vi "Get Dependencies.vi"(8 "error in (no error)":errorcluster, 11 "Instrument in":refnum<class "Instrument.lvclass">) -> (0 "error out":errorcluster, 2 "Dependencies":T1, 3 "Instrument out":refnum<class "Instrument.lvclass">)   [LabVIEW 2019, in "Instrument.lvlib" / "Instrument.lvclass"]
uses:
  Instrument.lvclass
  Typedefs/Dependencies--Cluster.ctl
  <userlib>/LevyLab/Configuration/Configuration.lvclass
  subsystems/HAL/HAL.lvclass
  subsystems/API/API.lvclass
  <userlib>/LevyLab/Logger.PGSQL/Logger.PGSQL/Logger.PGSQL.lvclass
  <userlib>/LevyLab/Logger.Error/Logger.Error/Logger.Error.lvclass
  <userlib>/LevyLab/RemoteControl/RemoteControl/RemoteControl.lvclass
  C:/Program Files (x86)/National Instruments/LabVIEW 2019/vi.lib/JKI/JKI SMO/SMO/SMO.lvclass
  Instrument.lvclass/Instrument.ctl
  Typedefs/Dependencies--Enum.ctl
  <vilib>/JKI/JKI SMO/SMO/SMO.lvclass
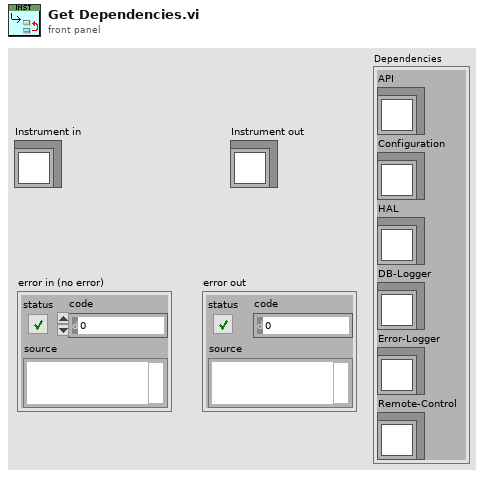
[diagram p1: front panel]
types:
  T1 = typedef "Instrument.lvlib/Instrument.lvclass/Dependencies--Cluster.ctl" = cluster{"API":refnum<class "API.lvclass">, "Configuration":refnum<class "Configuration.lvclass">, "HAL":refnum<class "HAL.lvclass">, "DB-Logger":refnum<class "Logger.PGSQL.lvclass">, "Error-Logger":refnum<class "Logger.Error.lvclass">, "Remote-Control":refnum<class "RemoteControl.lvclass">}
  T2 = typedef "Instrument.lvlib/Instrument.lvclass/Dependencies--Enum.ctl" = enum16{"API", "Configuration", "HAL", "DB-Logger", "Error-Logger", "Remote-Control"}
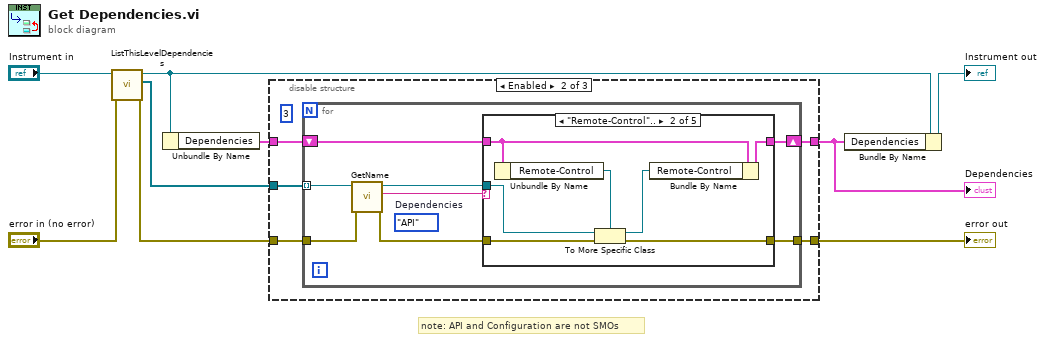
[diagram p0: block diagram]
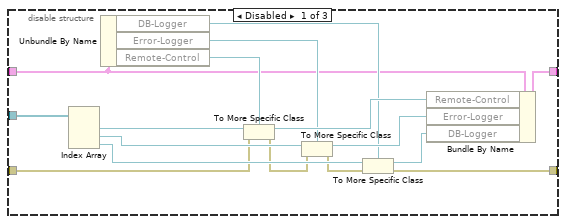
[diagram p2: hidden frame]
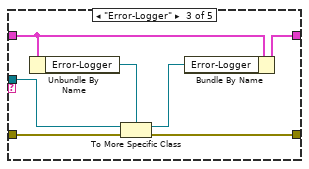
[diagram p4: hidden frame]
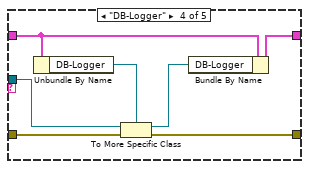
[diagram p5: hidden frame]
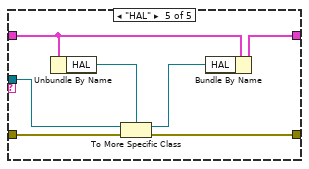
[diagram p6: hidden frame]
diagram:
  # "note: API and Configuration are not SMOs"
  n1 = call <vilib>:"ListThisLevelDependencies.vi"("error in (no error)"="error in (no error)", "SMO in"="Instrument in") -> ("error out"=w7:errorcluster, "[My Dependencies]"=w2:refnum<class "SMO.lvclass">[], "SMO out"=w5:refnum<class "Instrument.lvclass">)  [unwired: 7 in]
  n2 = Unbundle By Name(w5) -> ("Dependencies"=w4:T1)
  n3 = disable-structure shown="Enabled" {
    disable-tunnel: w7 -> [w20 w29 w69]
    disable-tunnel: w4 -> [w16 w26 w70]
    disable-tunnel: [w15 w28 w69] -> w3
    disable-tunnel: w2 -> [w14 w30 _]
    disable-tunnel: [w13 w27 w70] -> w1
    frame Disabled {
      n4 = Index Array(array=w14) -> (element #1=w25:refnum<class "SMO.lvclass">, element #2=w23:refnum<class "SMO.lvclass">, element #3=w22:refnum<class "SMO.lvclass">)  [unwired: 3 in]
      n5 = Unbundle By Name(w16) -> ("DB-Logger"=w17:refnum<class "Logger.PGSQL.lvclass">, "Error-Logger"=w18:refnum<class "Logger.Error.lvclass">, "Remote-Control"=w19:refnum<class "RemoteControl.lvclass">)
      n6 = To More Specific Class(target class=w19, reference=w25, error in=w20) -> (specific class reference=w24:refnum<class "RemoteControl.lvclass">, error out=w10:errorcluster)
      n7 = To More Specific Class(target class=w18, reference=w23, error in=w10) -> (specific class reference=w21:refnum<class "Logger.Error.lvclass">, error out=w11:errorcluster)
      n8 = To More Specific Class(target class=w17, reference=w22, error in=w11) -> (specific class reference=w12:refnum<class "Logger.PGSQL.lvclass">, error out=w15:errorcluster)
      n9 = Bundle By Name(cluster=w16, "Remote-Control"=w24, "Error-Logger"=w21, "DB-Logger"=w12) -> (w13:T1)
    }
    frame Enabled {
      (unwired) 3
      n10 = for {
        tunnel: w29 -> [w34]
        tunnel: [w37] -> w28
        shift-right: [w36] -> w27
        shift-left: w26 -> [w38]
        tunnel: w30 -> [w35] mode=indexing
        (unwired) Dependencies--Enum."API"  # Dependencies
        n11 = call <vilib>:"GetName.vi"("error in (no error)"=w34, "SMO"=w35) -> ("error out"=w33:errorcluster, "Name"=w31:string, "SMO out"=w32:refnum<class "SMO.lvclass">)  [unwired: 6 in, 1 out]
        n12 = case shown="\"Remote-Control\".." w31 {
          tunnel: w38 -> [w40 w47 w54 w61 w68]
          tunnel: [w39 w45 w52 w59 w66] -> w37
          tunnel: [w40 w44 w51 w58 w65] -> w36
          tunnel: w32 -> [_ w41 w48 w55 w62]
          tunnel: w33 -> [w39 w42 w49 w56 w63]
          frame Default {
          }
          frame "Remote-Control".. {
            n13 = Unbundle By Name(w47) -> ("Remote-Control"=w46:refnum<class "RemoteControl.lvclass">)
            n14 = To More Specific Class(target class=w46, reference=w41, error in=w42) -> (specific class reference=w43:refnum<class "RemoteControl.lvclass">, error out=w45:errorcluster)
            n15 = Bundle By Name(cluster=w47, "Remote-Control"=w43) -> (w44:T1)
          }
          frame "Error-Logger" {
            n16 = Unbundle By Name(w54) -> ("Error-Logger"=w53:refnum<class "Logger.Error.lvclass">)
            n17 = To More Specific Class(target class=w53, reference=w48, error in=w49) -> (specific class reference=w50:refnum<class "Logger.Error.lvclass">, error out=w52:errorcluster)
            n18 = Bundle By Name(cluster=w54, "Error-Logger"=w50) -> (w51:T1)
          }
          frame "DB-Logger" {
            n19 = Unbundle By Name(w61) -> ("DB-Logger"=w60:refnum<class "Logger.PGSQL.lvclass">)
            n20 = To More Specific Class(target class=w60, reference=w55, error in=w56) -> (specific class reference=w57:refnum<class "Logger.PGSQL.lvclass">, error out=w59:errorcluster)
            n21 = Bundle By Name(cluster=w61, "DB-Logger"=w57) -> (w58:T1)
          }
          frame "HAL" {
            n22 = Unbundle By Name(w68) -> ("HAL"=w67:refnum<class "HAL.lvclass">)
            n23 = To More Specific Class(target class=w67, reference=w62, error in=w63) -> (specific class reference=w64:refnum<class "HAL.lvclass">, error out=w66:errorcluster)
            n24 = Bundle By Name(cluster=w68, "HAL"=w64) -> (w65:T1)
          }
        }
      }
    }
    frame Disabled {
    }
  }
  "error out" <- w3
  "Dependencies" <- w1
  n25 = Bundle By Name(cluster=w5, "Dependencies"=w1) -> (→"Instrument out":refnum<class "Instrument.lvclass">)
